vi "HXGpid_popup.vi"(8 "error in (no error)":errorcluster) -> (0 "error out":errorcluster)   [LabVIEW 2012]
uses:
  Modules/PID/HXG2pid.ctl
  Controls/HXG2_AirPIDresets.ctl
  Controls/HXG2_LiqPIDresets.ctl
  PIDCtrl/HXG2_References.ctl
  Controls/HXG2_PIDgains_SchedulingArray_BasicBlock.ctl
  Controls/HXG2_PIDgains_SchedulingArray.ctl
  Controls/HXG2_PIDgains_SchedulingArrayWITHLimits.ctl
  Controls/HXG2_PIDgains_SchedulingRanges.ctl
panel:
  in  "SCHEDULE LIMITS":T1
  in  "PID":T2
  in  "LF PID Resets":T5
  in  "AF PID Resets":T6
  in  "Close":bool
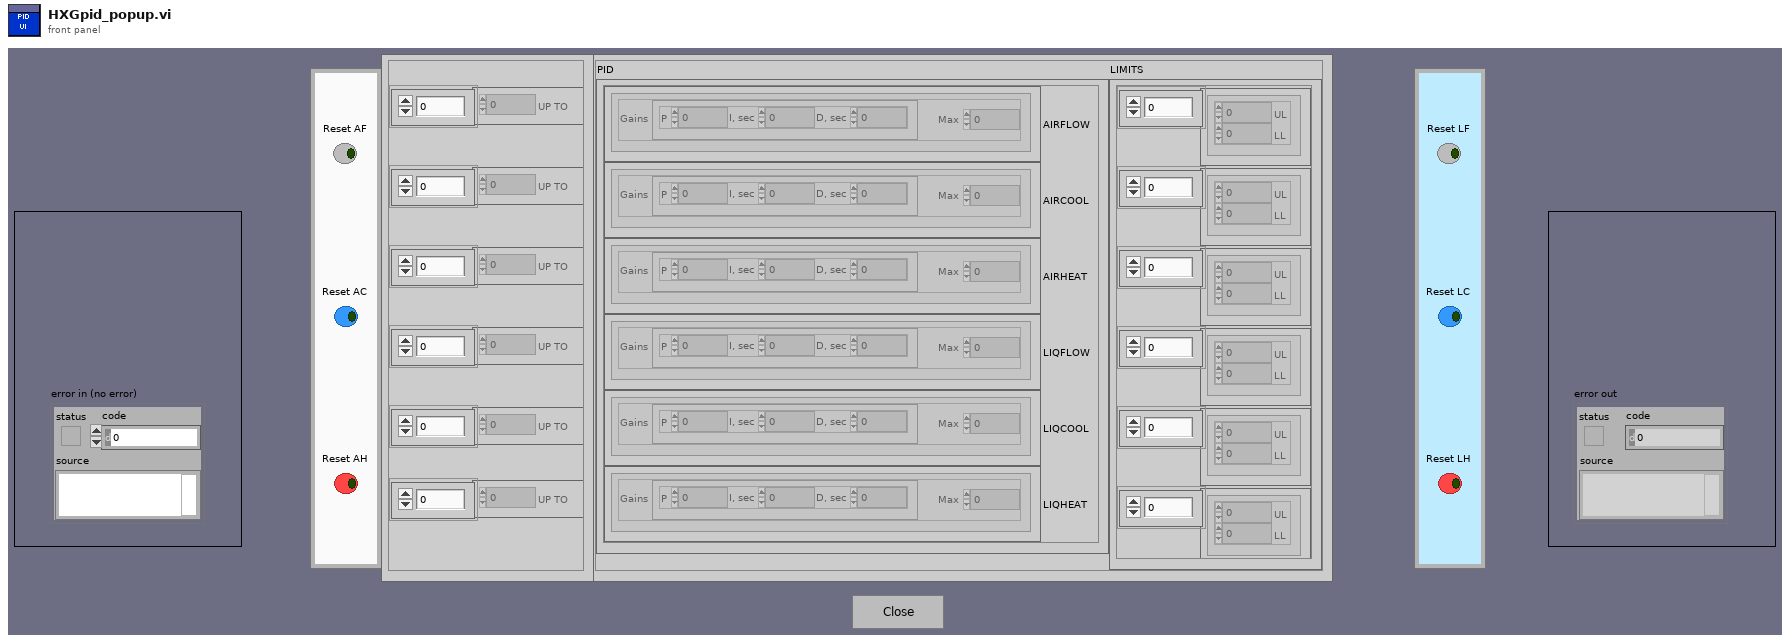
[diagram p1: front panel]
types:
  T1 = typedef "HXG2_PIDgains_SchedulingRanges.ctl" = cluster{"AIRFLOW 6":dbl[], "AIRFLOW 7":dbl[], "AIRFLOW 8":dbl[], "AIRFLOW 9":dbl[], "AIRFLOW 10":dbl[], "AIRFLOW 11":dbl[]}
  T2 = typedef "HXG2_PIDgains_SchedulingArrayWITHLimits.ctl" = cluster{"PID":T3, "LIMITS":cluster{"AIRFLOW":cluster{"UL":dbl, "LL  ":dbl}[], "AIRCOOL":cluster{"UL":dbl, "LL  ":dbl}[], "AIRHEAT":cluster{"UL":dbl, "LL  ":dbl}[], "LIQFLOW":cluster{"UL":dbl, "LL  ":dbl}[], "LIQCOOL":cluster{"UL":dbl, "LL  ":dbl}[], "LIQHEAT":cluster{"UL":dbl, "LL  ":dbl}[]}}
  T3 = typedef "HXG2_PIDgains_SchedulingArray.ctl" = cluster{"AIRFLOW":T4, "AIRCOOL":T4, "AIRHEAT":T4, "LIQFLOW":T4, "LIQCOOL":T4, "LIQHEAT":T4}
  T4 = typedef "HXG2_PIDgains_SchedulingArray_BasicBlock.ctl" = cluster{"Gains":cluster{"P":dbl, "I, sec":dbl, "D, sec":dbl}, "Max":dbl}[]
  T5 = typedef "HXG2_LiqPIDresets.ctl" = cluster{"Reset LF":bool, "Reset LC":bool, "Reset LH":bool}
  T6 = typedef "HXG2_AirPIDresets.ctl" = cluster{"Reset AF":bool, "Reset AC":bool, "Reset AH":bool}
  T7 = typedef "HXG2pid.ctl" = enum16{"Write PID Efforts", "Write PID On-Off", "Pass", "Write PID Refs", "Write PID pop-up", "Wrt PID Resets"}
  T8 = typedef "HXG2_Horizontal PID Control.ctl" = cluster{"SchedLimsArray":cluster{"LL  ":dbl, "UL":dbl}[], "GainsArray":cluster{"Gains":cluster{"P":dbl, "I, sec":dbl, "D, sec":dbl}, "Max\nOutput":dbl}[], "UL-LL Array":cluster{"UL":dbl, "LL  ":dbl}[]}[]
  T9 = typedef "HXG2_References.ctl" = cluster{"AF PID ON":refnum<vi>, "AT PID ON":refnum<vi>, "LT PID ON":refnum<vi>, "LF PID ON":refnum<vi>, "Reset Ctrls":refnum<vi>[]}
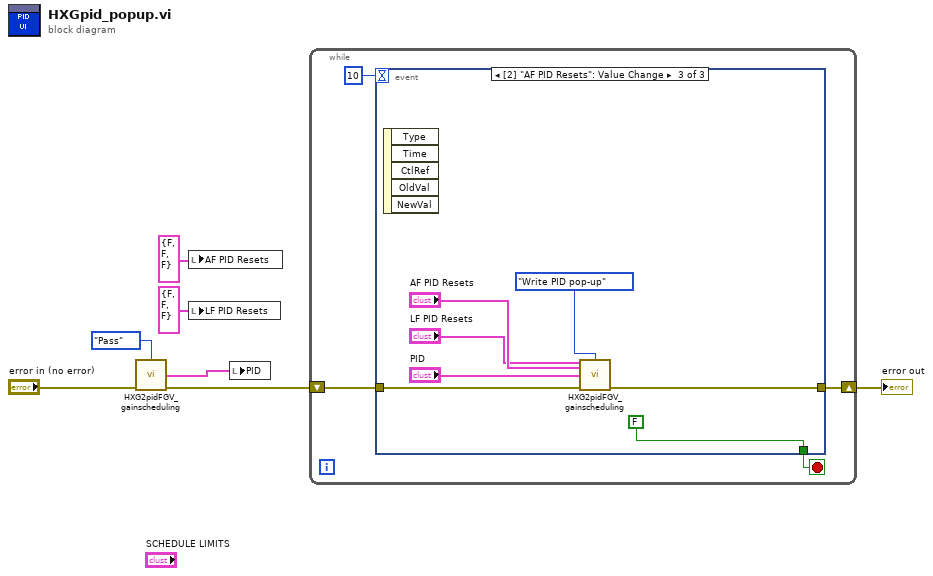
[diagram p0: block diagram]
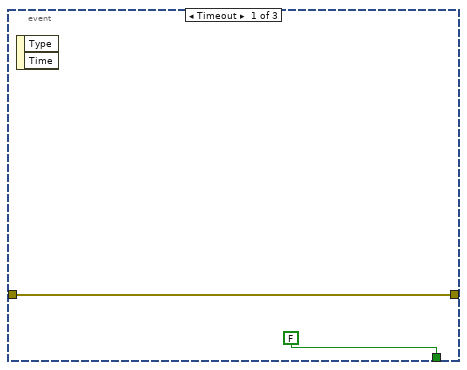
[diagram p2: hidden frame]
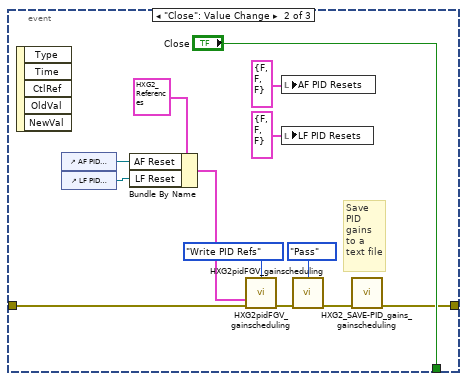
[diagram p3: hidden frame]
diagram:
  n1 = call "HXG2pidFGV_gainscheduling.vi"("PIDfgvCtrl"=HXG2pid."Pass", "error in (no error)"="error in (no error)") -> ("PID Gains Out"=w1:T8, "error out"=w5:errorcluster)  [unwired: 8 in, 4 out]
  n2 = local write "AF PID Resets"(T6 {"Reset AF"=FALSE, "Reset AC"=FALSE, "Reset AH"=FALSE} ("AF PID Resets")) -> ()
  n3 = local write "LF PID Resets"(T5 {"Reset LF"=FALSE, "Reset LC"=FALSE, "Reset LH"=FALSE} ("LF PID Resets")) -> ()
  n4 = local write "PID"(w1) -> ()
  n5 = while {
    shift-right: [w8] -> w7
    shift-left: w5 -> [w9]
    stop <- w10 stop-if-true
    n6 = event shown="[2] \"AF PID Resets\": Value Change" {
      selector: _ -> [_ _ _]
      dyn-events: _ -> [_ _ _]
      timeout: 10 -> [_ _ _]
      tunnel: [FALSE ("Cancel") "Close" FALSE ("Cancel")] -> w10
      tunnel: w9 -> [w13 w19 w32]
      tunnel: [w13 w25 w31] -> w8
      event Timeout {
        n7 = event-data() -> ()  [unwired: 1 in, 2 out]
      }
      event "Close": Value Change {
        # "Save PID gains \nto a text file"
        n8 = event-data() -> ()  [unwired: 1 in, 5 out]
        n9 = control-ref of="AF PID Resets"() -> (w15:refnum<vi>)
        n10 = control-ref of="LF PID Resets"() -> (w14:refnum<vi>)
        n11 = Bundle By Name(cluster=T9 {"AF PID ON"=refnum, "AT PID ON"=refnum, "LT PID ON"=refnum, "LF PID ON"=refnum, "Reset Ctrls"=[]} ("PID Ref cluster"), "AF Reset"=w15, "LF Reset"=w14) -> (w16:T9)
        n12 = call "HXG2pidFGV_gainscheduling.vi"("PIDfgvCtrl"=HXG2pid."Write PID Refs", "PID Ref cluster"=w16, "error in (no error)"=w19) -> ("error out"=w20:errorcluster)  [unwired: 7 in, 5 out]
        n13 = local write "AF PID Resets"(T6 {"Reset AF"=FALSE, "Reset AC"=FALSE, "Reset AH"=FALSE} ("AF PID Resets")) -> ()
        n14 = local write "LF PID Resets"(T5 {"Reset LF"=FALSE, "Reset LC"=FALSE, "Reset LH"=FALSE} ("LF PID Resets")) -> ()
        n15 = call "HXG2pidFGV_gainscheduling.vi"("PIDfgvCtrl"=HXG2pid."Pass", "error in (no error)"=w20) -> ("error out"=w24:errorcluster)  [unwired: 8 in, 5 out]
        n16 = call "HXG2_SAVE-PID_gains_gainscheduling.vi"("error in"=w24) -> ("error out"=w25:errorcluster)  [unwired: 10 in]
      }
      event Value Change {
        n17 = event-data() -> ()  [unwired: 1 in, 5 out]
        n18 = call "HXG2pidFGV_gainscheduling.vi"(0:"LF PID Resets", "Reset PIDs"="AF PID Resets", "PIDfgvCtrl"=HXG2pid."Write PID pop-up", "PID gains in"="PID", "error in (no error)"=w32) -> ("error out"=w31:errorcluster)  [unwired: 5 in, 5 out]
      }
    }
  }
  "error out" <- w7
